vi "SENS_IF_FILT_ERR.vi"(0 "VISA IN":refnum<visa-resource-name>, 5 "error in":errorcluster, 7 "Channel":i32) -> (14 "VISA Out":refnum<visa-resource-name>, 16 "Data":string, 19 "error out":errorcluster)   [LabVIEW 2018, in "PNA-X.lvlib"]
doc: "SENSe<cnum>:IF:FILTer:ERRors? \n(Read-only) Returns the error string associated with the digital filters. The return string has three fields \nseparated by commas: \"stage1 status, stage2 status, stage3 status\" \nEach of these fields can contain one or more of the following error codes: \nNO ERROR \n*NUMBER-OF-COEFFICIENTS - the number of coefficients is excessive for that filter-stage \n*COEFFICIENT VALUE - one or more coefficients are out of range for that filter-stage \n*SUM-OF-COEFFICIENTS - the sum of all coefficients is excessive for that filter-stage, \n*FREQUENCY - the frequency for Stage 1 is out of range (only applies stage1 field), \n*PARAMETER - one or more parameters are out of range (only applies to stage 3 field) \nCritical Note \nParameters \n<cnum> Existing channel number. If unspecified, <cnum> is set to 1. \nExamples SENS:IF:FILT:ERR? \n'example return strings\" \nNO ERROR, NO ERROR, NO ERROR \nindicates no errors, \n*SUM-OF-COEFFICIENTS, NO ERROR, NO ERROR \nindicates that the sum of all filter coefficients exceed the \nmaximum value for the Stage-1 filter, \n*COEFFICIENT *SUM-OF-COEFFICIENTS, NO ERROR, *PARAMETER \nindicates a problems with Stage 1 coefficients and a problem with \none or more of the parameters associated with the Stage 3 filter. \nReturn Type String \nDefault Not Applicable"
uses:
  PNA-X.lvlib
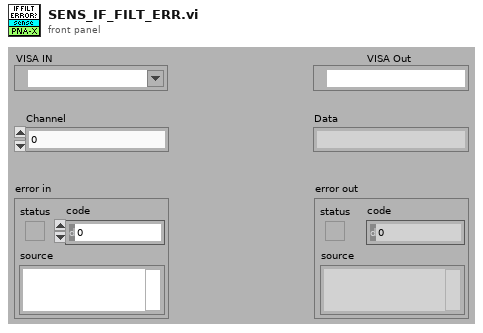
[diagram p1: front panel]
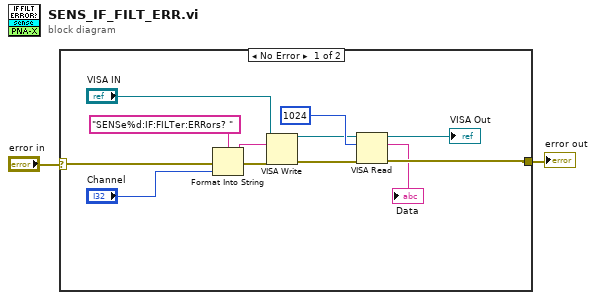
[diagram p0: block diagram]
diagram:
  n1 = case shown="No Error" "error in" {
    selector: "error in" -> [w14 w15]
    tunnel: [w5 w15] -> w1
    frame No Error {
      n2 = Format Into String(format string="SENSe%d:IF:FILTer:ERRors? " ("Cmdline"), error in=w14, "Channel") -> (resulting string=w12:string, error out=w13:errorcluster)  [unwired: 1 in]
      n3 = VISA Write(VISA resource name="VISA IN", write buffer=w12, error in (no error)=w13) -> (VISA resource name out=w7:refnum<visa-resource-name>, error out=w9:errorcluster)  [unwired: 1 out]
      n4 = VISA Read(VISA resource name=w7, byte count=1024, error in (no error)=w9) -> (VISA resource name out=→"VISA Out":refnum<visa-resource-name>, read buffer=→"Data":string, error out=w5:errorcluster)  [unwired: 1 out]
    }
    frame Error {
    }
  }
  "error out" <- w1
